vi "Find pos limit mMc.vi"(1 "Port":T1={"P type"=0, "reference"="", " Terminator "="\r\n", "Timeout"=300} {"Timeout" step=10; "P type" items=["none", "RS-232C"]}, 2 "timeout":u32=30000, 3 "error in (no error)":errorcluster, 5 "Controller #":string) -> (7 "timeout?":bool, 9 "error out":errorcluster)   [LabVIEW 2013]
panel:
  # "Find positive travel limit"
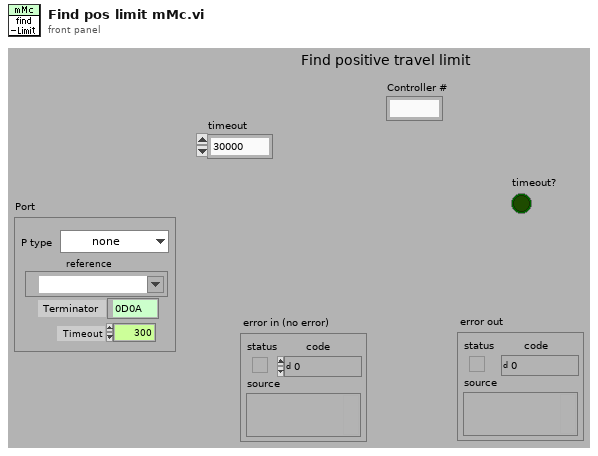
[diagram p1: front panel]
types:
  T1 = cluster{"P type":u16, "reference":refnum<visa-resource-name>, " Terminator ":string, "Timeout":i32}
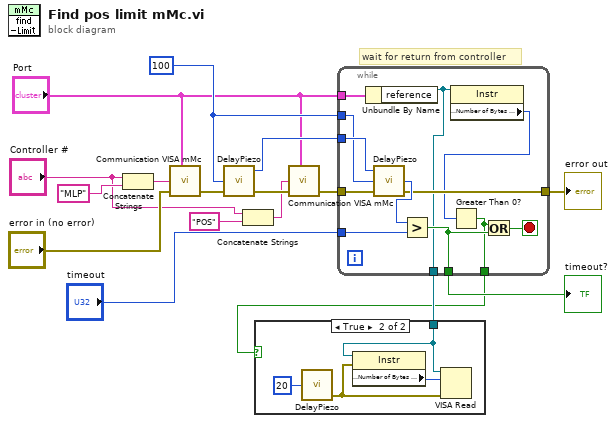
[diagram p0: block diagram]
diagram:
  w12 = u32 100 ("milliseconds to wait")
  # "wait for return from controller"
  n1 = Concatenate Strings("Controller #", "MLP") -> (w15:string)
  n2 = call "Communication VISA mMc.vi"("Port"="Port", "Command"=w15, "error in (no error)"="error in (no error)") -> ("error out"=w14:errorcluster)  [unwired: 3 in, 3 out]
  n3 = call "DelayPiezo.vi"("milliseconds to wait"=w12, "error in (no error)"=w14) -> ("new time"=w13:u32, "error out"=w6:errorcluster)  [unwired: 5 in, 1 out]
  n4 = Concatenate Strings("Controller #", "POS") -> (w3:string)
  n5 = call "Communication VISA mMc.vi"("Port"="Port", "Command"=w3, "error in (no error)"=w6) -> ("error out"=w5:errorcluster)  [unwired: 3 in, 3 out]
  n6 = while {
    tunnel: w5 -> [w29]
    tunnel: "Port" -> [w21]
    tunnel: w13 -> [w28]
    tunnel: w12 -> [w25]
    tunnel: [w22] -> w11
    tunnel: [w24] -> w10
    tunnel: "timeout" -> [w23]
    tunnel: [w20] -> w8
    tunnel: [w18] -> w7
    stop <- w26 stop-if-true
    n7 = Unbundle By Name(w21) -> ("reference"=w20:refnum<visa-resource-name>)
    n8 = call "DelayPiezo.vi"("old timer value"=w28, "milliseconds to wait"=w25, "error in (no error)"=w29) -> ("elapsed time"=w27:u32, "error out"=w22:errorcluster)  [unwired: 4 in, 1 out]
    n9 = Greater?(x=w27, y=w23) -> (0:w24:bool)
    n10 = property class="Instr"(reference=w20) -> ("Serial Settings:Number of Bytes at Serial Port"=w19:u32)  [unwired: 1 in, 2 out]
    n11 = Greater Than 0?(x=w19) -> (x > 0?=w18:bool)
    n12 = Or(x=w18, y=w24) -> (x .or. y?=w26:bool)
  }
  "error out" <- w11
  "timeout?" <- w10
  n13 = case shown="True" w7 {
    tunnel: w8 -> [_ w32]
    frame False {
    }
    frame True {
      n14 = call "DelayPiezo.vi"("milliseconds to wait"=u32 20) -> ("error out"=w33:errorcluster)  [unwired: 6 in, 2 out]
      n15 = property class="Instr"(reference=w32, error in=w33) -> ("Serial Settings:Number of Bytes at Serial Port"=w31:u32)  [unwired: 2 out]
      n16 = VISA Read(VISA resource name=w32, byte count=w31, error in (no error)=w33) -> ()  [unwired: 4 out]
    }
  }
